vi "Numeric_to_boolean.vi"(5 "Numeric":i32) -> (2 "Bool":bool)   [LabVIEW 2010]
doc: "Converts a numeric (I32) to boolean. 0: false, everything else: true."
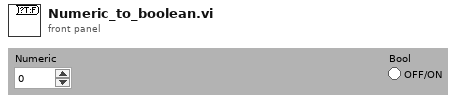
[diagram p1: front panel]
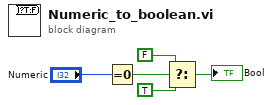
[diagram p0: block diagram]
diagram:
  n1 = Equal To 0?(x="Numeric") -> (x = 0?=w4:bool)
  n2 = Select(t=FALSE, s=w4, f=TRUE) -> (s? t:f=→"Bool":bool)
